vi "PQprotocolVersion.vi"(8 "error in (no error)":errorcluster, 10 "conn":u64) -> (0 "error out":errorcluster, 3 "PQprotocolVersion":u64)   [LabVIEW 2019, in "libpqlv64.lvlib"]
doc: "Interrogates the frontend/backend protocol being used."
uses:
  libpqlv64.lvlib
  libpq.dll
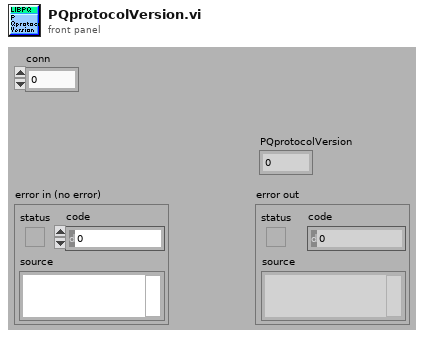
[diagram p1: front panel]
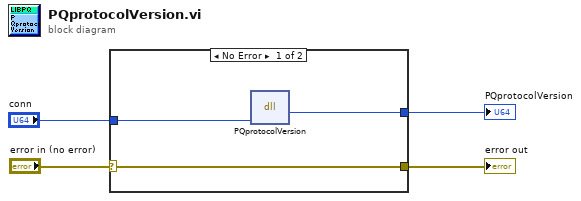
[diagram p0: block diagram]
diagram:
  n1 = case shown="No Error" "error in (no error)" {
    selector: "error in (no error)" -> [w7 w8]
    tunnel: [w7 w8] -> w3
    tunnel: [w6 _] -> w2
    tunnel: "conn" -> [w5 _]
    frame No Error {
      n2 = dll-call lib="libpq.*" fn="PQprotocolVersion"("conn"=w5) -> ("PQprotocolVersion"=w6:u64)  [unwired: 4 in, 2 out]
    }
    frame Error {
    }
  }
  "PQprotocolVersion" <- w2
  "error out" <- w3
